vi "lord_Read_Off_Gain_All_Chx_v2.vi"(0 "CCS":T1={"Port Number"=1444, "Core Number"=1, "Page"=0}, 5 "lv_ref_sel":u16, 7 "lv_ref_vol":u16, 9 "lv_scomp":u16=8, 11 "error in":errorcluster, 12 "VREF":dbl=3.3) -> (2 "Mean[]":dbl[](array[numeric]), 3 "Range[]":u16[](array[numeric]) format="%#.0f", 4 "CCS out":T1={"Port Number"=1444, "Core Number"=1, "Page"=0}, 6 "Min[]":u16[](array[numeric]) format="%#.0f", 8 "appended array":dbl[][](array[numeric]), 10 "Max[]":u16[](array[numeric]) format="%#.0f", 13 "Channel Names":string[](array[string])=["ADC0_Chx0_PA27_pin31x", "ADC0_Chx1_PA26_pin30x", "ADC0_Chx2_PA25_pin29x", "ADC0_Chx3_PA24_pin28x", "ADC0_Chx4_PA22_pin26x", "ADC0_Chx5_PA21_pin25xREFM", "ADC0_Chx6_PA20_pin24x", "ADC0_Chx7_PA18_pin22x", "ADC0_Chx8_PA16_pin20x", "ADC0_Chx9_PA15_pin19x", "ADC0_Chx10_INT_pinxUNBUFpad", "ADC0_Chx11_INT_pinxTEMPSNS", "ADC0_Chx12_INT_pinxOPA0out", "ADC0_Chx13_INT_pinxOPA1out", "ADC0_Chx14_INT_pinxGPAMPout", "ADC0_Chx15_INT_pinxVDDSNS"], 14 "SD[]":dbl[](array[numeric]), 15 "error out":errorcluster={"status"=TRUE, "code"=1, "source"="TCP Write in CCS.lvlib:Get Symbol Address.vi:3380045->CCS.lvlib:Write Data To Symbol - U16.vi:5420008->lord_Read_Off_Gain_All_Chx_v2.vi"})   [LabVIEW 2019]
uses:
  <userlib>/_TI-LA/Reusable/CCS/APIs/Data/Polymorphics/Write Data To Symbol - U16.vi
  <userlib>/_TI-LA/Reusable/CCS/APIs/Data/Polymorphics/Read Data From Symbol - U16 Array.vi
  <userlib>/_TI-LA/Reusable/CCS/APIs/Data/Polymorphics/Read Data From Symbol - Float Array.vi
  <userlib>/_TI-LA/Reusable/CCS/APIs/CCS.lvlib
panel:
  out "Mean_V":dbl[](array[numeric])
  out "LSB(V)":dbl format="%#_3p"
  # "uint16_t lv_ref_sel     =   0; //0=vdda, 1=extref, 2=intref\nuint16_t lv_ref_vol     =   0; //0=2P5V, 1=1P4V\nuint16_t lv_scomp       =   8; //8Clocks of 32M give = 250ns"
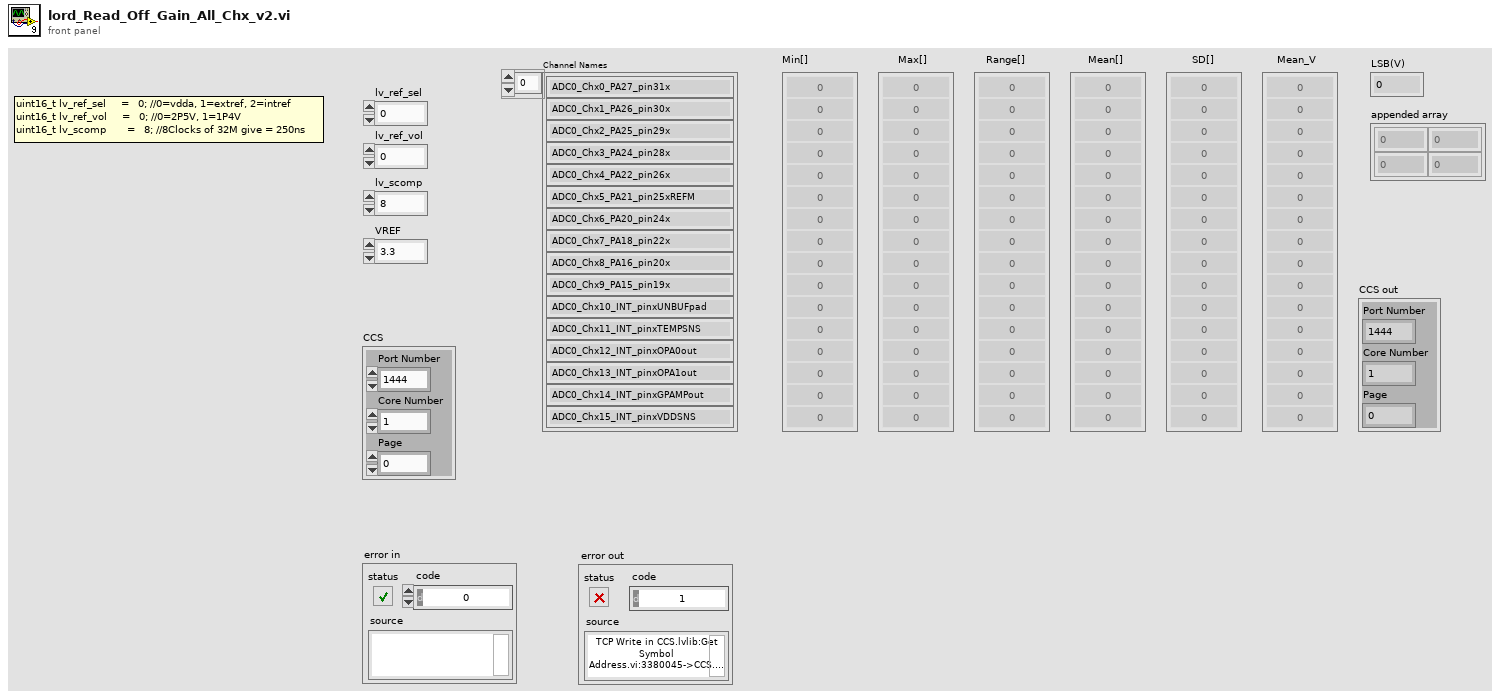
[diagram p1: front panel]
types:
  T1 = cluster{"Port Number":u16, "Core Number":u16, "Page":i32}
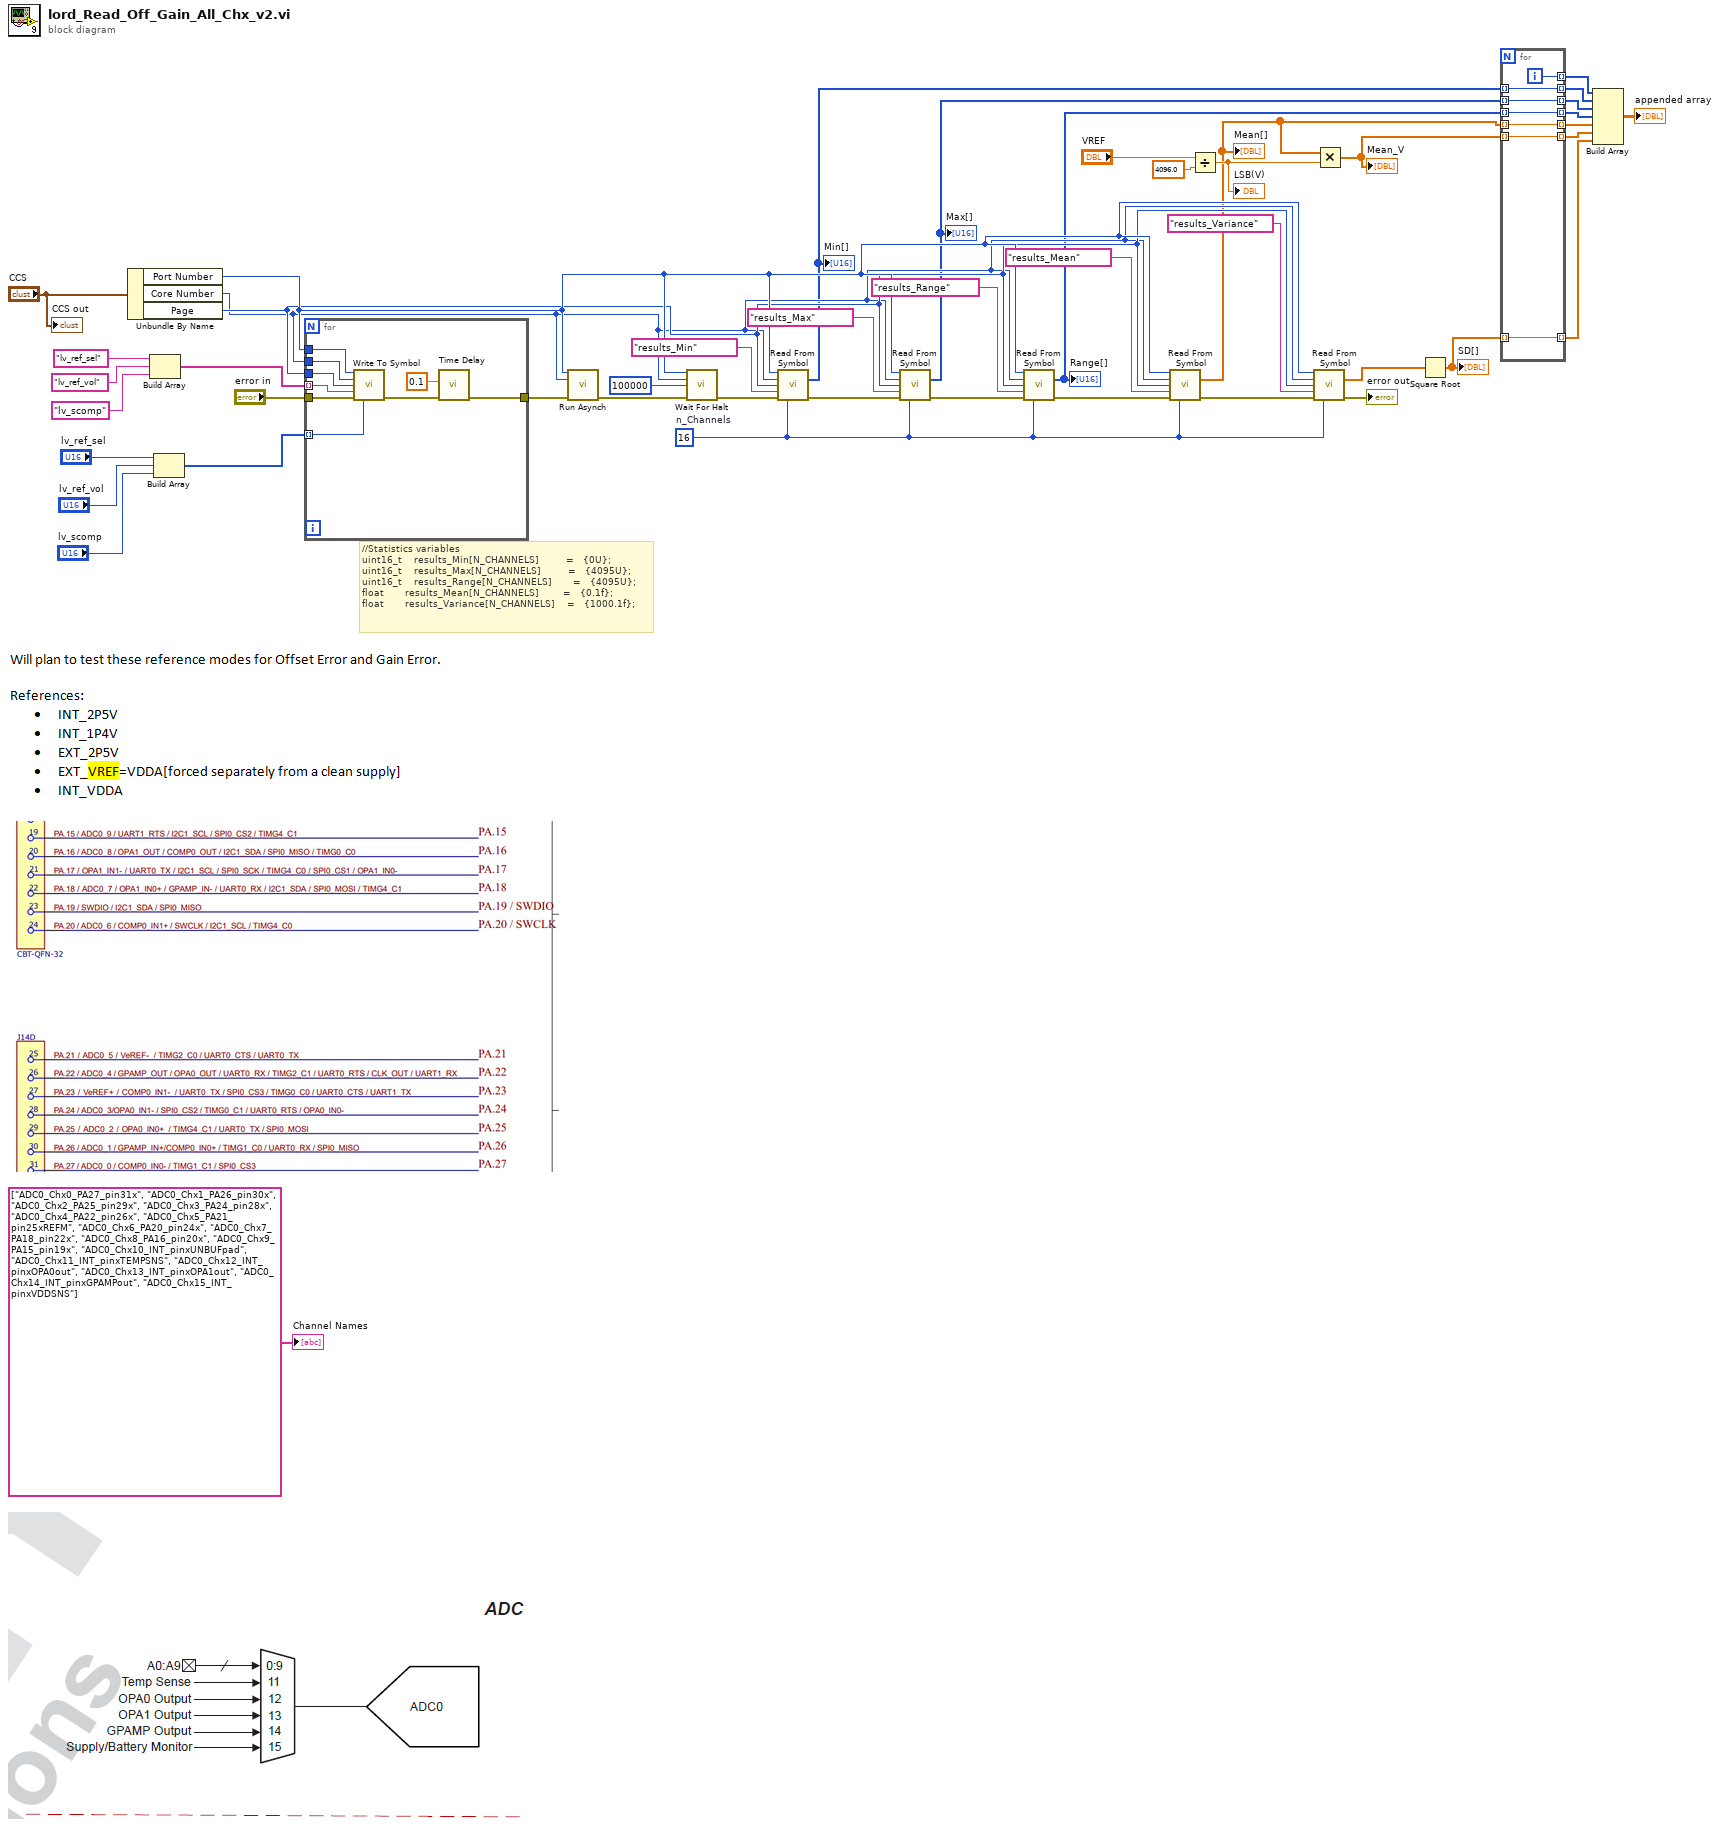
[diagram p0: block diagram]
diagram:
  w36 = u32 16  # n_Channels
  # "//Statistics variables\nuint16_t    results_Min[N_CHANNELS]         =   {0U};\nuint16_t    results_Max[N_CHANNELS]         =   {4095U};\nuint16_t    results_Range[N_CHANNELS]       =   {4095U};\nfloat       results_Mean[N_CHANNELS]        =   {0.1f};\nfloat       results_Variance[N_CHANNELS]    =   {1000.1f};"
  n1 = Unbundle By Name("CCS") -> ("Port Number"=w26:u16, "Core Number"=w24:u16, "Page"=w25:i32)
  n2 = Build Array("lv_ref_sel", "lv_ref_vol", "lv_scomp") -> (w30:string[])
  n3 = Build Array("lv_ref_sel", "lv_ref_vol", "lv_scomp") -> (w31:u16[])
  n4 = for {
    tunnel: w30 -> [w56] mode=indexing
    tunnel: w31 -> [w54] mode=indexing
    tunnel: [w53] -> w29
    tunnel: w25 -> [w51]
    tunnel: w26 -> [w50]
    tunnel: w24 -> [w49]
    tunnel: "error in" -> [w48]
    n5 = call-poly <userlib>:"Write To Symbol.vi"("Port Number"=w50, "Core Number"=w49, "Page"=w51, "Symbol Name"=w56, "error in"=w48, "Write Data"=w54) -> ("error out"=w55:errorcluster)  [unwired: 7 in, 2 out]
    n6 = call "Time Delay"("error in (no error)"=w55, "Delay Time (s)"=0.1) -> ("error out"=w53:errorcluster)  [unwired: 9 in]
  }
  n7 = call <userlib>:"Run Asynch.vi"("Port Number"=w26, "Core Number"=w24, "error in"=w29) -> ("error out"=w33:errorcluster)  [unwired: 10 in, 2 out]
  n8 = call <userlib>:"Wait For Halt.vi"("Port Number"=w26, "Core Number"=w24, "Timeout (10k)(ms)"=100000, "error in"=w33) -> ("error out"=w28:errorcluster)  [unwired: 9 in, 2 out]
  n9 = call-poly <userlib>:"Read From Symbol.vi"("Port Number"=w26, "Core Number"=w24, "Page"=w25, "Symbol Name"="results_Min", "error in"=w28, "Data Length"=w36) -> ("Read Data[]"=w13:u16[], "error out"=w47:errorcluster)  [unwired: 6 in, 2 out]
  "Min[]" <- w13
  n10 = call-poly <userlib>:"Read From Symbol.vi"("Port Number"=w26, "Core Number"=w24, "Page"=w25, "Symbol Name"="results_Max", "error in"=w47, "Data Length"=w36) -> ("Read Data[]"=w10:u16[], "error out"=w46:errorcluster)  [unwired: 6 in, 2 out]
  "Max[]" <- w10
  n11 = call-poly <userlib>:"Read From Symbol.vi"("Port Number"=w26, "Core Number"=w24, "Page"=w25, "Symbol Name"="results_Range", "error in"=w46, "Data Length"=w36) -> ("Read Data[]"=w8:u16[], "error out"=w45:errorcluster)  [unwired: 6 in, 2 out]
  "Range[]" <- w8
  n12 = call-poly <userlib>:"Read From Symbol.vi"("Port Number"=w26, "Core Number"=w24, "Page"=w25, "Symbol Name"="results_Mean", "error in"=w45, "Data Length"=w36) -> ("Read Data[]"=w6:dbl[], "error out"=w44:errorcluster)  [unwired: 6 in, 2 out]
  "Mean[]" <- w6
  n13 = Divide(x="VREF", y=4096.0) -> (x/y=w21:dbl)
  "LSB(V)" <- w21
  n14 = call-poly <userlib>:"Read From Symbol.vi"("Port Number"=w26, "Core Number"=w24, "Page"=w25, "Symbol Name"="results_Variance", "error in"=w44, "Data Length"=w36) -> ("Read Data[]"=w43:dbl[], "error out"=→"error out":errorcluster)  [unwired: 6 in, 2 out]
  n15 = Multiply(x=w6, y=w21) -> (x*y=w4:dbl[])
  "Mean_V" <- w4
  n16 = Square Root(x=w43) -> (sqrt(x)=w2:dbl[])
  "SD[]" <- w2
  n17 = for {
    tunnel: [w63] -> w14 mode=indexing
    tunnel: w13 -> [w63] mode=indexing
    tunnel: [w62] -> w12 mode=indexing
    tunnel: [w61] -> w11 mode=indexing
    tunnel: w10 -> [w61] mode=indexing
    tunnel: [w60] -> w9 mode=indexing
    tunnel: w8 -> [w60] mode=indexing
    tunnel: [w59] -> w7 mode=indexing
    tunnel: w6 -> [w59] mode=indexing
    tunnel: [w58] -> w5 mode=indexing
    tunnel: w4 -> [w58] mode=indexing
    tunnel: [w57] -> w3 mode=indexing
    tunnel: w2 -> [w57] mode=indexing
    i -> [w62]
  }
  n18 = Build Array(w12, w14, w11, w9, w7, w5, w3) -> (→"appended array":dbl[][])
  "CCS out" <- "CCS"
  "Channel Names" <- string[] ["ADC0_Chx0_PA27_pin31x", "ADC0_Chx1_PA26_pin30x", "ADC0_Chx2_PA25_pin29x", "ADC0_Chx3_PA24_pin28x", "ADC0_Chx4_PA22_pin26x", "ADC0_Chx5_PA21_pin25xREFM", "ADC0_Chx6_PA20_pin24x", "ADC0_Chx7_PA18_pin22x", "ADC0_Chx8_PA16_pin20x", "ADC0_Chx9_PA15_pin19x", "ADC0_Chx10_INT_pinxUNBUFpad", "ADC0_Chx11_INT_pinxTEMPSNS", "ADC0_Chx12_INT_pinxOPA0out", "ADC0_Chx13_INT_pinxOPA1out", "ADC0_Chx14_INT_pinxGPAMPout", "ADC0_Chx15_INT_pinxVDDSNS"]
